vi "AMI_Queue_Commands.vi"(1 "AMI_Control":T1, 2 "Last Status":T1, 3 "Queue in":refnum<queue>) -> (0 "New Status":T1)   [LabVIEW 2018]
uses:
  AMI/AMI_Control.ctl
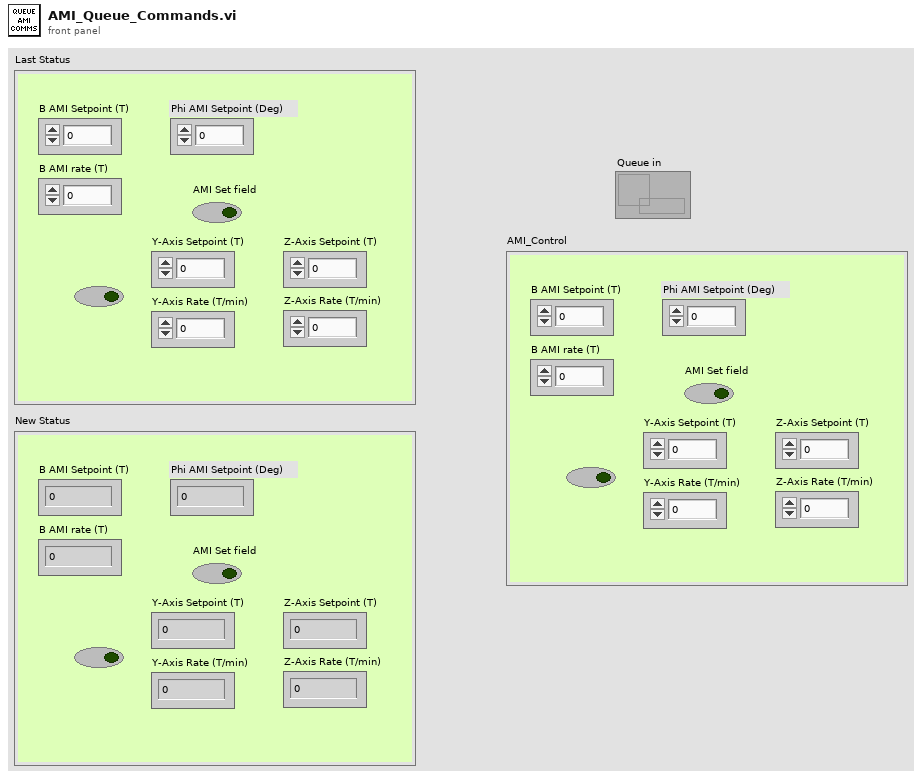
[diagram p1: front panel]
types:
  T1 = typedef "AMI_Control.ctl" = cluster{"B AMI rate (T)":dbl, "AMI Set field":bool, "B AMI Setpoint (T)":dbl, "Phi AMI Setpoint (Deg) ":dbl, "Switch Heater":bool, "Y-Axis Setpoint (T)":dbl, "Y-Axis Rate (T/min)":dbl, "Z-Axis Setpoint (T)":dbl, "Z-Axis Rate (T/min)":dbl}
  T2 = cluster{"B AMI rate (T)":bool, "AMI Set field":bool, "B AMI Setpoint (T)":bool, "Phi AMI Setpoint (Deg) ":bool, "Switch Heater":bool, "Y-Axis Setpoint (T)":bool, "Y-Axis Rate (T/min)":bool, "Z-Axis Setpoint (T)":bool, "Z-Axis Rate (T/min)":bool}
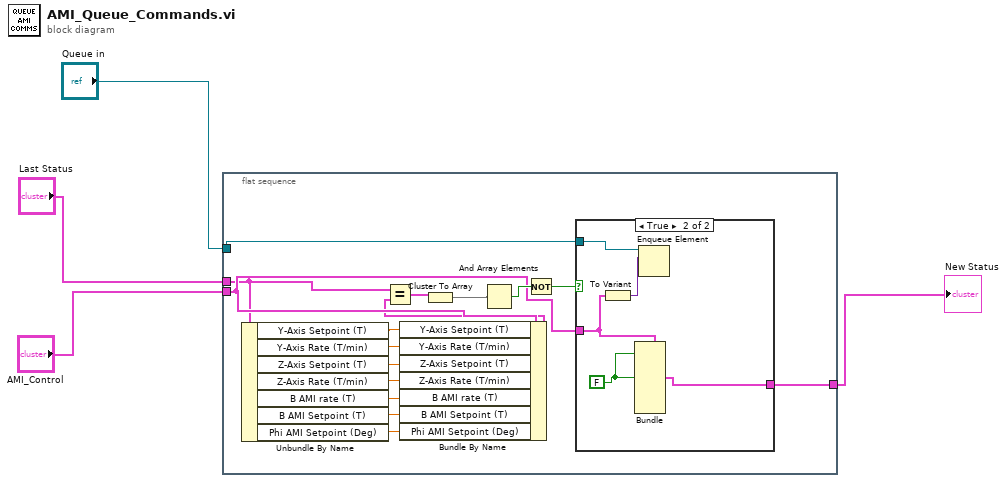
[diagram p0: block diagram]
diagram:
  n1 = flat-sequence {
    tunnel: "Queue in" -> [w20]
    tunnel: "AMI_Control" -> [w14]
    tunnel: "Last Status" -> [w12]
    tunnel: [w15] -> w1
    frame #0 {
      n2 = Unbundle By Name(w12) -> ("Y-Axis Setpoint (T)"=w11:dbl, "Y-Axis Rate (T/min)"=w10:dbl, "Z-Axis Setpoint (T)"=w9:dbl, "Z-Axis Rate (T/min)"=w8:dbl, "B AMI rate (T)"=w7:dbl, "B AMI Setpoint (T)"=w6:dbl, "Phi AMI Setpoint (Deg)"=w5:dbl)
      n3 = Bundle By Name(cluster=w14, "Y-Axis Setpoint (T)"=w11, "Y-Axis Rate (T/min)"=w10, "Z-Axis Setpoint (T)"=w9, "Z-Axis Rate (T/min)"=w8, "B AMI rate (T)"=w7, "B AMI Setpoint (T)"=w6, "Phi AMI Setpoint (Deg)"=w5) -> (w13:T1)
      n4 = Equal?(x=w12, y=w13) -> (x = y?=w16:T2)
      n5 = Cluster To Array(cluster=w16) -> (array=w19:bool[])
      n6 = And Array Elements(Boolean array=w19) -> (logical AND=w18:bool)
      n7 = Not(x=w18) -> (.not. x?=w17:bool)
      n8 = case shown="True" w17 {
        tunnel: w20 -> [_ w26]
        tunnel: w14 -> [w21 w24]
        tunnel: [w21 w23] -> w15
        frame False {
        }
        frame True {
          w22 = FALSE
          n9 = To Variant(anything=w24) -> (Variant=w25:variant)
          n10 = Bundle(cluster=w24, "AMI Set field"=w22, "Switch Heater"=w22) -> (w23:T1)  [unwired: 7 in]
          n11 = Enqueue Element(queue=w26, element=w25) -> ()  [unwired: 2 in, 3 out]
        }
      }
    }
  }
  "New Status" <- w1
